vi "set Current.vi"(10 "curr":sgl, 11 "devID":u32) -> (3 "function return":i32)   [LabVIEW 2014, in "libchaos-driver-powersupply-labview.lvlib"]
doc: "int setCurrent(unsigned int devID,float curr);"
uses:
  libchaos-driver-powersupply-labview.lvlib
  chaos-i686-dynamic-release/lib/libchaos-driver-powersupply-labview.so
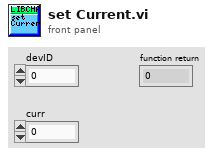
[diagram p1: front panel]
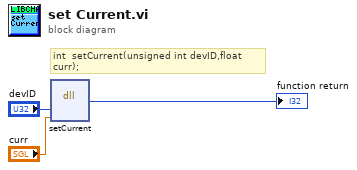
[diagram p0: block diagram]
diagram:
  # "int  setCurrent(unsigned int devID,float curr);"
  n1 = dll-call lib="home/chaos/chaos_bundle/chaos-i686-dynamic-release/lib/libchaos-driver-powersupply-labview.*" fn="setCurrent"("devID"="devID", "curr"="curr") -> (→"function return":i32)  [unwired: 5 in, 2 out]
